vi "UTFencoder.vi"(10 "LabVIEW string":string) -> (2 "UTF-8 string":string)   [LabVIEW 2015, in "AWS_IoT.lvlib"]
uses:
  AWS_IoT.lvlib
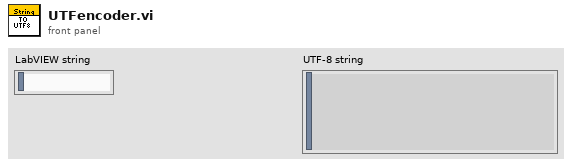
[diagram p1: front panel]
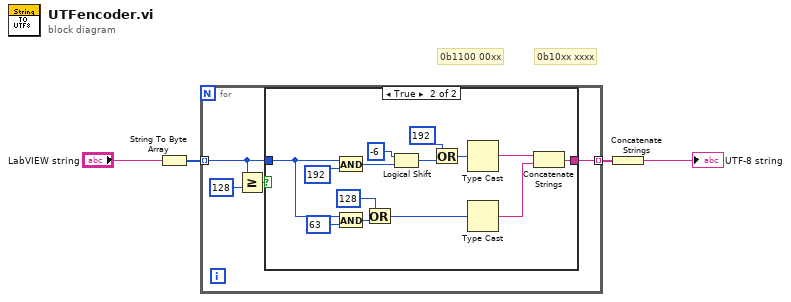
[diagram p0: block diagram]
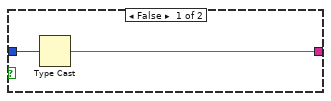
[diagram p2: hidden frame]
diagram:
  # "0b10xx xxxx"
  # "0b1100 00xx"
  n1 = String To Byte Array(string="LabVIEW string") -> (unsigned byte array=w3:u8[])
  n2 = for {
    tunnel: w3 -> [w6] mode=indexing
    tunnel: [w5] -> w4 mode=indexing
    n3 = Greater Or Equal?(x=w6, y=u8 128) -> (x >= y?=w7:bool)
    n4 = case shown="True" w7 {
      tunnel: w6 -> [w10 w23]
      tunnel: [w9 w13] -> w5
      frame False {
        n5 = Type Cast(x=w10) -> (*(type *) &x=w9:string)  [unwired: 1 in]
      }
      frame True {
        n6 = And(x=w23, y=u8 192) -> (x .and. y?=w21:u8)
        n7 = And(x=w23, y=u8 63) -> (x .and. y?=w19:u8)
        n8 = Or(x=u8 128 ("y"), y=w19) -> (x .or. y?=w14:u8)
        n9 = Logical Shift(y=i16 -6, x=w21) -> (x << y=w17:u8)
        n10 = Or(x=u8 192 ("y"), y=w17) -> (x .or. y?=w15:u8)
        n11 = Type Cast(x=w15) -> (*(type *) &x=w12:string)  [unwired: 1 in]
        n12 = Type Cast(x=w14) -> (*(type *) &x=w11:string)  [unwired: 1 in]
        n13 = Concatenate Strings(w12, w11) -> (w13:string)
      }
    }
  }
  n14 = Concatenate Strings(w4) -> (→"UTF-8 string":string)
